vi "Main.vi"() -> ()   [LabVIEW 2014]
uses:
  Temp Sensor Folder/Global Stop TempSensor.vi
  StopForLog.vi
panel:
  out "Path":path
  out "User Name 2":string caption="שם משתמש"
  out "מספר סידורי 2":string caption="מספר סידורי"
  in  "בחירה חופשית":bool caption="Blank Button"
  in  "ממסר השהייה למפוח מפנה גזים 0410-26308":bool caption="Blank Button"
  in  "ממסר דימום מנוע 0410-26294":bool caption="Blank Button"
  in  "0410-24534 15A ממסר":bool caption="Blank Button"
  in  "0410-19646 10Ax4 ממסר":bool caption="Blank Button"
  in  "תיבת נתיכים סימן 4 0414-83040":bool caption="Blank Button"
  in  "תיבת מפעיל ריצוף 1469-98836":bool caption="Blank Button"
  in  "תיבת הזנה כיס צריח 0410-23813":bool caption="Blank Button"
  in  "Help Button":bool
  in  "Stop Button":bool
  # "צב\"ד לממסרים ונתיכים"
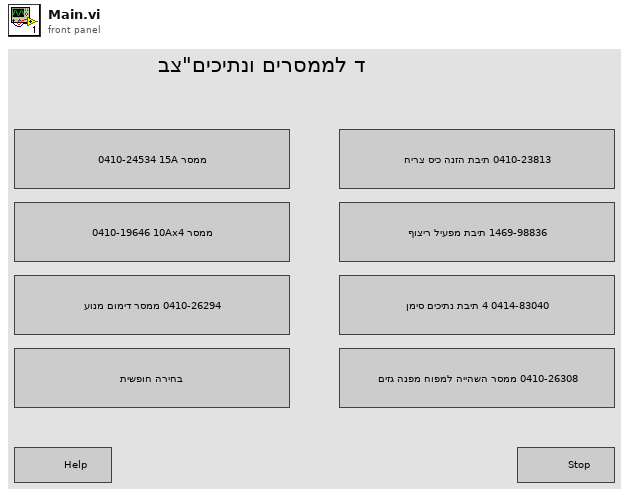
[diagram p1: front panel]
types:
  T1 = enum16{"Word Report", "User/Details", "Stop", "bhira hofshit", "ashaya mapuah mefane gazim 041026308", "dimum manoa 041026294", "memsar 4x10A 041019646", "memsar 15A 041024534", "netihim siman 4 041483040", "mafil risouf 146998836", "kis zariah 041023813", "Wait4Event", "Initialize"}
  T2 = enum16{"open", "replace", "create", "open or create", "replace or create", "replace or create with confirmation"}
  T3 = enum32{"Invalid", "Standard", "Closed", "Hidden", "Minimized", "Maximized"}
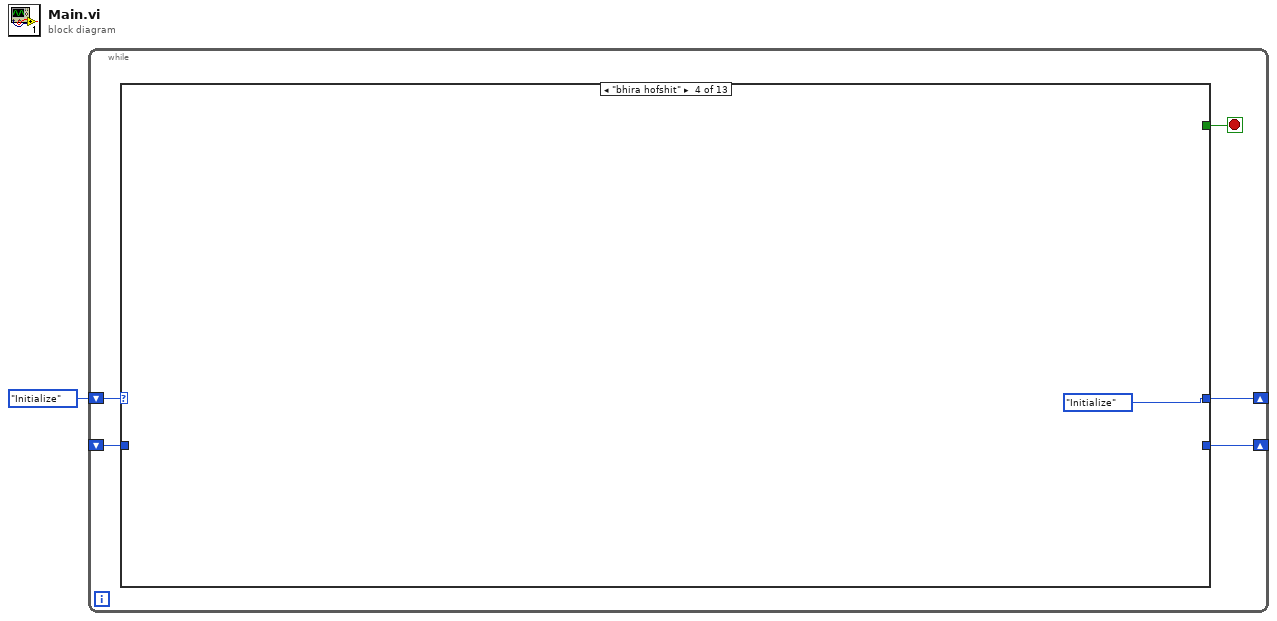
[diagram p0: block diagram]
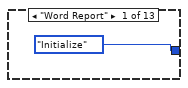
[diagram p2: hidden frame]
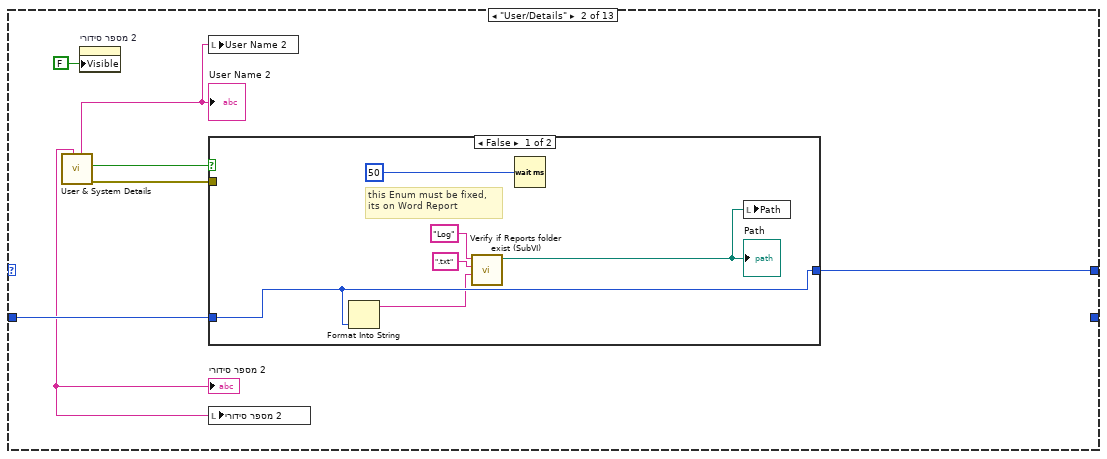
[diagram p3: hidden frame]
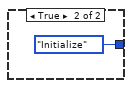
[diagram p4: hidden frame]
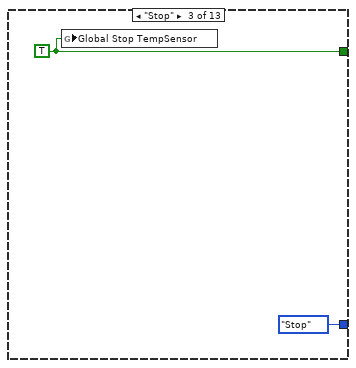
[diagram p5: hidden frame]
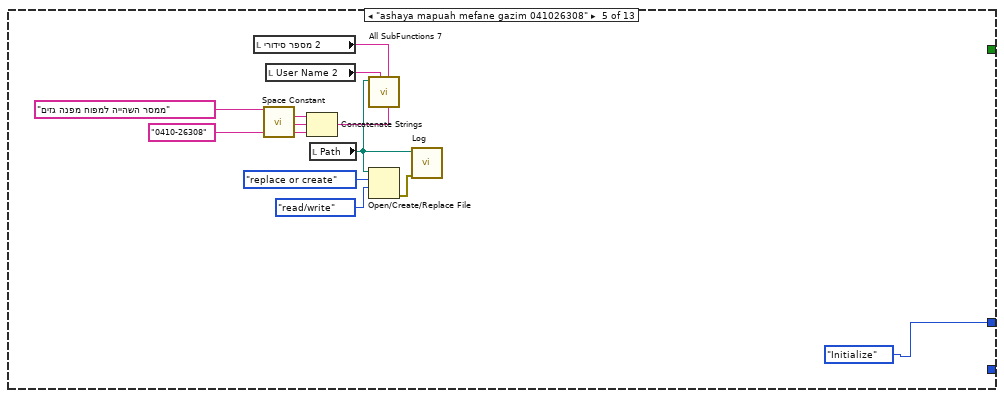
[diagram p6: hidden frame]
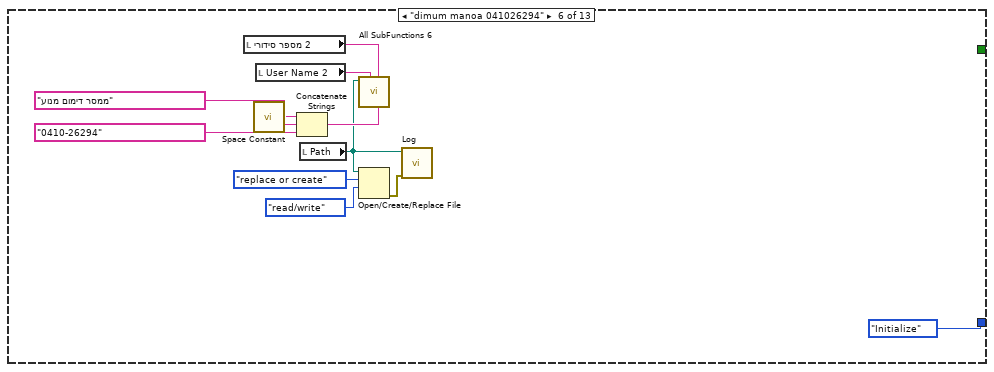
[diagram p7: hidden frame]
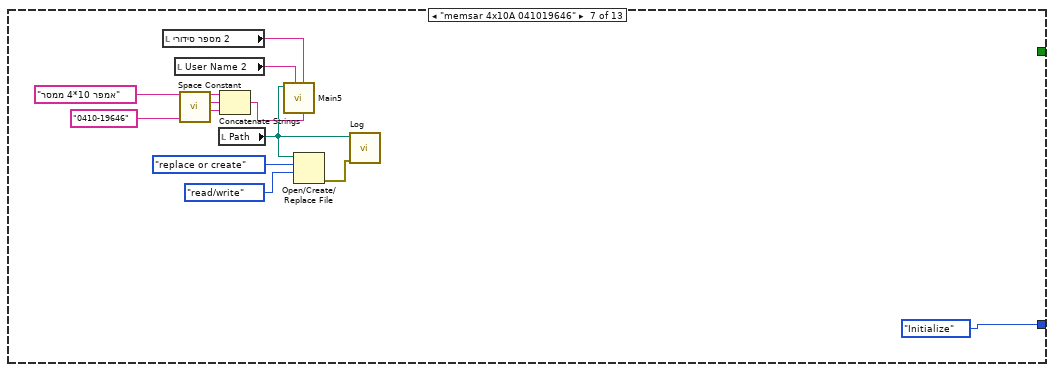
[diagram p8: hidden frame]
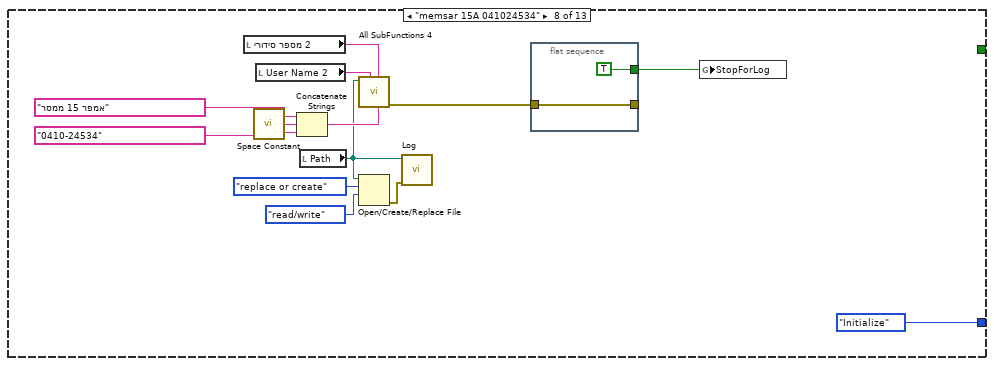
[diagram p9: hidden frame]
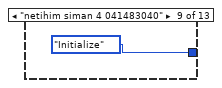
[diagram p10: hidden frame]
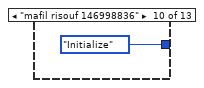
[diagram p11: hidden frame]
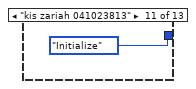
[diagram p12: hidden frame]
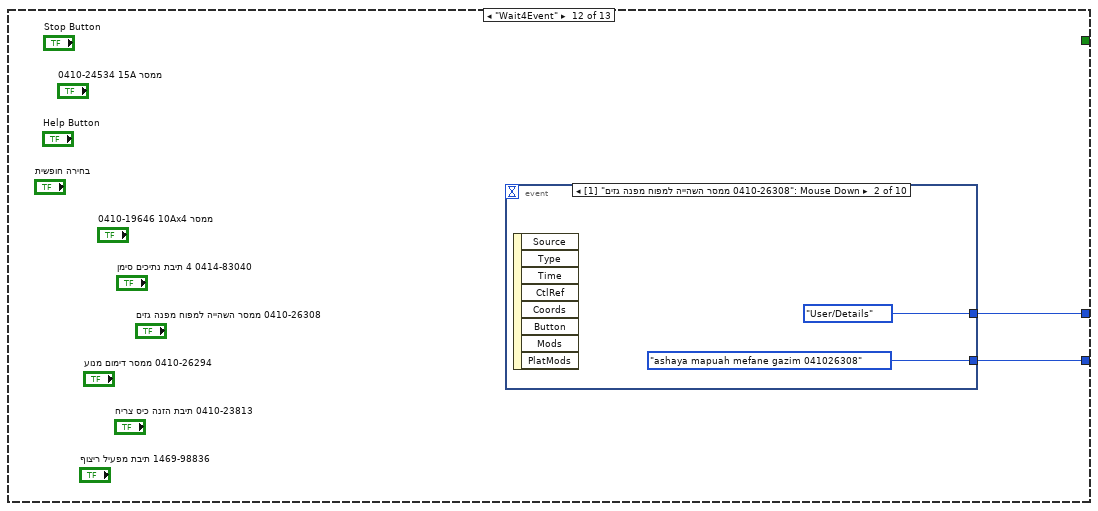
[diagram p13: hidden frame]
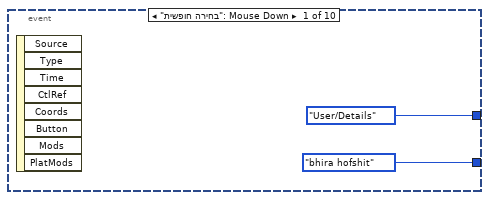
[diagram p14: hidden frame]
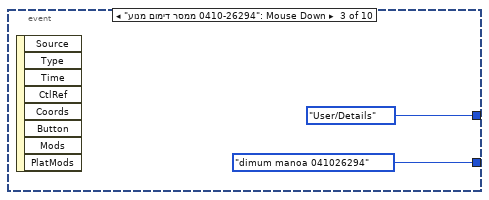
[diagram p15: hidden frame]
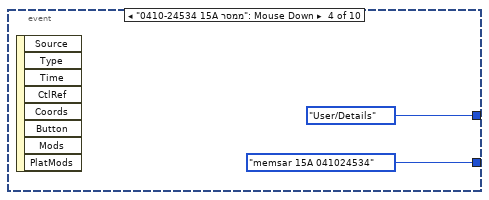
[diagram p16: hidden frame]
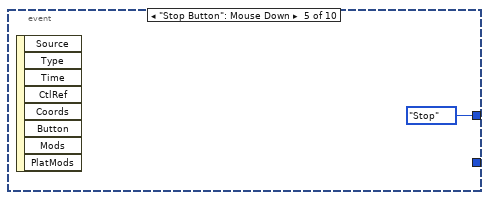
[diagram p17: hidden frame]
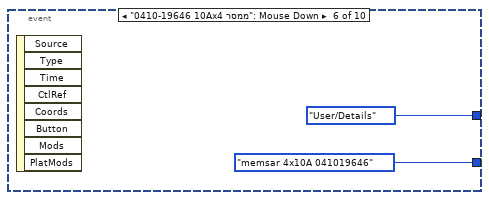
[diagram p18: hidden frame]
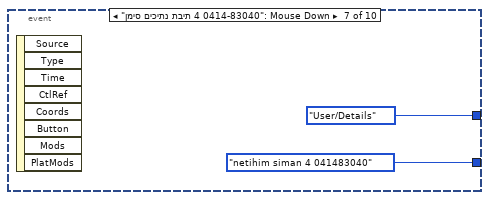
[diagram p19: hidden frame]
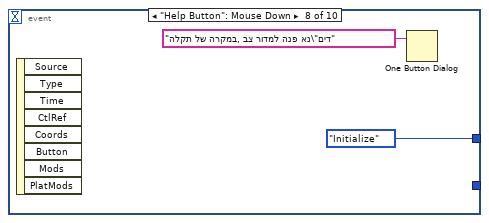
[diagram p20: hidden frame]
diagram:
  n1 = while {
    shift-right: [w5] -> _
    shift-left: T1."Initialize" -> [w6]
    shift-right: [w3] -> _
    shift-left: _ -> [w2]
    stop <- w4 stop-if-true
    n2 = case shown="\"bhira hofshit\"" w6 {
      tunnel: [T1."Initialize" w8 T1."Stop" T1."Initialize" T1."Initialize" T1."Initialize" T1."Initialize" T1."Initialize" T1."Initialize" T1."Initialize" T1."Initialize" w77 T1."Wait4Event"] -> w5
      tunnel: [_ _ w22 _ _ _ _ _ _ _ _ _ _] -> w4
      tunnel: [_ _ _ _ _ _ _ _ _ _ _ w76 _] -> w3
      tunnel: w2 -> [_ w13 _ _ _ _ _ _ _ _ _ _ _]
      frame "Word Report" {
      }
      frame "User/Details" {
        n3 = call "User & System Details.vi"() -> ("error out"=w12:errorcluster, "Boolean"=w14:bool, "User Name 2"=w9:string, "מספר סידורי 2"=w11:string)  [unwired: 8 in]
        "מספר סידורי 2" <- w11
        "User Name 2" <- w9
        n4 = property on="מספר סידורי 2" class="Str"("Visible"=FALSE) -> ()  [unwired: 2 in, 2 out]
        n5 = local write "User Name 2"(w9) -> ()
        n6 = case shown="False" w14 {
          tunnel: w13 -> [w16 _]
          tunnel: w12 -> [_ _]
          tunnel: [w16 T1."Initialize"] -> w8
          frame False {
            # "this Enum must be fixed, \nits on Word Report"
            n7 = Format Into String "Format Into String"(w16) -> (resulting string=w15:string)  [unwired: 3 in, 1 out]
            n8 = call "Verify if Reports folder exist (SubVI).vi"("שם הממסר"=w15, "File Type"=".txt", "Folder Name"="Log" ("string")) -> ("Path"=w17:path)  [unwired: 7 in, 1 out]
            "Path" <- w17
            n9 = Wait (ms)(milliseconds to wait=u32 50) -> ()  [unwired: 1 out]
            n10 = local write "Path"(w17) -> ()
          }
          frame True {
          }
        }
        n11 = local write "מספר סידורי 2"(w11) -> ()
      }
      frame "Stop" {
        w22 = TRUE
        n12 = global write "Global Stop TempSensor.vi" "Global Stop TempSensor"(w22) -> ()
      }
      frame "bhira hofshit" {
      }
      frame "ashaya mapuah mefane gazim 041026308" {
        n13 = local read "מספר סידורי 2"() -> (w31:string)
        n14 = call <vilib>:"Space Constant.vi"() -> ("String"=w34:string)
        n15 = local read "User Name 2"() -> (w32:string)
        n16 = Concatenate Strings("ממסר השהייה למפוח מפנה גזים", w34, "0410-26308") -> (w35:string)
        n17 = local read "Path"() -> (w26:path)
        n18 = call "All SubFunctions 7.vi"("מק\"ט המכלל"=w35, "מספר סידורי"=w31, "מפעיל"=w32, "Path for Log"=w26) -> ()  [unwired: 7 in, 1 out]
        n19 = Open/Create/Replace File(file path (use dialog)=w26, operation (0:open)=T2."replace or create", access (0:read/write)=enum16{"read/write", "read-only", "write-only"}."read/write") -> (error out=w27:errorcluster)  [unwired: 3 in, 2 out]
        n20 = call "Log.vi"("error in"=w27, "File Path Control"=w26) -> ()  [unwired: 8 in, 2 out]
      }
      frame "dimum manoa 041026294" {
        n21 = local read "מספר סידורי 2"() -> (w38:string)
        n22 = call <vilib>:"Space Constant.vi"() -> ("String"=w46:string)
        n23 = local read "User Name 2"() -> (w37:string)
        n24 = Concatenate Strings("ממסר דימום מנוע", w46, "0410-26294") -> (w41:string)
        n25 = local read "Path"() -> (w39:path)
        n26 = call "All SubFunctions 6.vi"("מק\"ט המכלל"=w41, "מספר סידורי"=w38, "מפעיל"=w37, "Path for Log"=w39) -> ()  [unwired: 7 in, 1 out]
        n27 = Open/Create/Replace File(file path (use dialog)=w39, operation (0:open)=T2."replace or create", access (0:read/write)=enum16{"read/write", "read-only", "write-only"}."read/write") -> (error out=w40:errorcluster)  [unwired: 3 in, 2 out]
        n28 = call "Log.vi"("error in"=w40, "File Path Control"=w39) -> ()  [unwired: 8 in, 2 out]
      }
      frame "memsar 4x10A 041019646" {
        n29 = local read "מספר סידורי 2"() -> (w48:string)
        n30 = local read "User Name 2"() -> (w49:string)
        n31 = call <vilib>:"Space Constant.vi"() -> ("String"=w55:string)
        n32 = local read "Path"() -> (w50:path)
        n33 = Concatenate Strings("ממסר 4*10 אמפר", w55, "0410-19646") -> (w52:string)
        n34 = call "Main5.vi"("מק\"ט המכלל"=w52, "מספר סידורי"=w48, "מפעיל"=w49, "Path for Log"=w50) -> ()  [unwired: 7 in, 1 out]
        n35 = Open/Create/Replace File(file path (use dialog)=w50, operation (0:open)=T2."replace or create", access (0:read/write)=enum16{"read/write", "read-only", "write-only"}."read/write") -> (error out=w51:errorcluster)  [unwired: 3 in, 2 out]
        n36 = call "Log.vi"("error in"=w51, "File Path Control"=w50) -> ()  [unwired: 8 in, 2 out]
      }
      frame "memsar 15A 041024534" {
        n37 = local read "מספר סידורי 2"() -> (w59:string)
        n38 = call <vilib>:"Space Constant.vi"() -> ("String"=w64:string)
        n39 = local read "User Name 2"() -> (w58:string)
        n40 = Concatenate Strings("ממסר 15 אמפר", w64, "0410-24534") -> (w66:string)
        n41 = local read "Path"() -> (w60:path)
        n42 = call "All SubFunctions 4.vi"("מק\"ט המכלל"=w66, "מספר סידורי"=w59, "מפעיל"=w58, "Path for Log"=w60) -> ("error IO"=w62:errorcluster)  [unwired: 7 in]
        n43 = Open/Create/Replace File(file path (use dialog)=w60, operation (0:open)=T2."replace or create", access (0:read/write)=enum16{"read/write", "read-only", "write-only"}."read/write") -> (error out=w63:errorcluster)  [unwired: 3 in, 2 out]
        n44 = call "Log.vi"("error in"=w63, "File Path Control"=w60) -> ()  [unwired: 8 in, 2 out]
        n45 = flat-sequence {
          tunnel: w62 -> [w71]
          tunnel: [TRUE] -> w61
          tunnel: [w71] -> _
          frame #0 {
          }
        }
        n46 = global write "StopForLog.vi" "StopForLog"(w61) -> ()
      }
      frame "netihim siman 4 041483040" {
      }
      frame "mafil risouf 146998836" {
      }
      frame "kis zariah 041023813" {
      }
      frame "Wait4Event" {
        n47 = event shown="[1] \"ממסר השהייה למפוח מפנה גזים 0410-26308\": Mouse Down" {
          selector: _ -> [_ _ _ _ _ _ _ _ _ _]
          dyn-events: _ -> [_ _ _ _ _ _ _ _ _ _]
          timeout: _ -> [_ _ _ _ _ _ _ _ _ _]
          tunnel: [T1."User/Details" T1."User/Details" T1."User/Details" T1."User/Details" T1."Stop" T1."User/Details" T1."User/Details" T1."Initialize" T1."User/Details" T1."User/Details"] -> w77
          tunnel: [T1."bhira hofshit" T1."ashaya mapuah mefane gazim 041026308" T1."dimum manoa 041026294" T1."memsar 15A 041024534" _ T1."memsar 4x10A 041019646" T1."netihim siman 4 041483040" _ T1."mafil risouf 146998836" T1."kis zariah 041023813"] -> w76
          event "בחירה חופשית": Mouse Down {
            n48 = event-data() -> ()  [unwired: 1 in, 8 out]
          }
          event "ממסר השהייה למפוח מפנה גזים 0410-26308": Mouse Down {
            n49 = event-data() -> ()  [unwired: 1 in, 8 out]
          }
          event "ממסר דימום מנוע 0410-26294": Mouse Down {
            n50 = event-data() -> ()  [unwired: 1 in, 8 out]
          }
          event "0410-24534 15A ממסר": Mouse Down {
            n51 = event-data() -> ()  [unwired: 1 in, 8 out]
          }
          event "Stop Button": Mouse Down {
            n52 = event-data() -> ()  [unwired: 1 in, 8 out]
          }
          event "0410-19646 10Ax4 ממסר": Mouse Down {
            n53 = event-data() -> ()  [unwired: 1 in, 8 out]
          }
          event "תיבת נתיכים סימן 4 0414-83040": Mouse Down {
            n54 = event-data() -> ()  [unwired: 1 in, 8 out]
          }
          event "Help Button": Mouse Down {
            n55 = event-data() -> ()  [unwired: 1 in, 8 out]
            n56 = One Button Dialog(message="במקרה של תקלה, נא פנה למדור צב\"דים") -> ()  [unwired: 1 in, 1 out]
          }
          event "תיבת מפעיל ריצוף 1469-98836": Mouse Down {
            n57 = event-data() -> ()  [unwired: 1 in, 8 out]
          }
          event "תיבת הזנה כיס צריח 0410-23813": Mouse Down {
            n58 = event-data() -> ()  [unwired: 1 in, 8 out]
          }
        }
      }
      frame "Initialize", Default {
        n59 = vi-ref "Main.vi"() -> (w99:refnum<vi>)
        n60 = global write "Global Stop TempSensor.vi" "Global Stop TempSensor"(FALSE ("Global Stop TempSensor")) -> ()
        n61 = property class="VI"(reference=w99) -> (reference out=w98:refnum<vi>, "FP.State"=w97:T3)  [unwired: 1 in, 1 out]
        n62 = case shown="\"Closed\"" w97 {
          tunnel: w98 -> [w111 w113 w117 w119 w123 w125]
          frame "Invalid", Default {
            n63 = invoke class="VI" method="FP.Open"(reference=w111, "Activate"=FALSE ("Wait Until Done"), "State"=T3."Standard") -> ()  [unwired: 2 in, 5 out]
          }
          frame "Standard" {
            n64 = invoke class="VI" method="FP.Open"(reference=w113, "Activate"=FALSE ("Wait Until Done"), "State"=T3."Standard") -> ()  [unwired: 2 in, 5 out]
          }
          frame "Closed" {
            n65 = invoke class="VI" method="FP.Open"(reference=w117, "Activate"=FALSE ("Wait Until Done"), "State"=T3."Standard") -> ()  [unwired: 2 in, 5 out]
          }
          frame "Hidden" {
            n66 = invoke class="VI" method="FP.Open"(reference=w119, "Activate"=FALSE ("Wait Until Done"), "State"=T3."Standard") -> ()  [unwired: 2 in, 5 out]
          }
          frame "Minimized" {
            n67 = invoke class="VI" method="FP.Open"(reference=w123, "Activate"=FALSE ("Wait Until Done"), "State"=T3."Standard") -> ()  [unwired: 2 in, 5 out]
          }
          frame "Maximized" {
            n68 = invoke class="VI" method="FP.Open"(reference=w125, "Activate"=FALSE ("Wait Until Done"), "State"=T3."Standard") -> ()  [unwired: 2 in, 5 out]
          }
        }
        n69 = call <vilib>:"Application Directory.vi"() -> ("Application Directory"=w108:path)
        n70 = Build Path(base path=w108, name or relative path="Temp Sensor Folder\\Temp Sensor.vi") -> (appended path=w106:path)
        n71 = Open VI Reference(vi path=w106) -> (vi reference=w105:refnum<vi>, error out=w104:errorcluster)  [unwired: 5 in]
        n72 = property class="VI"(reference=w105, error in=w104) -> (reference out=w101:refnum<vi>, error out=w102:errorcluster, "FP.State"=w103:T3)
        n73 = case shown="\"Invalid\", Default" w103 {
          tunnel: w102 -> [w129 w136 w142 _ _ _]
          tunnel: w101 -> [w128 w135 w143 _ _ _]
          frame "Invalid", Default {
            w134 = FALSE ("Wait Until Done")
            n74 = invoke class="VI" method="FP.Open"(reference=w128, error in=w129, "Activate"=w134, "State"=T3."Minimized") -> (reference out=w131:refnum<vi>, error out=w132:errorcluster)  [unwired: 1 in, 3 out]
            n75 = invoke class="VI" method="Run VI"(reference=w131, error in=w132, "Wait until done"=w134, "Auto Dispose Ref"=FALSE ("Auto Dispose Reference")) -> ()  [unwired: 1 in, 5 out]
          }
          frame "Standard" {
            w141 = FALSE ("Wait Until Done")
            n76 = invoke class="VI" method="FP.Open"(reference=w135, error in=w136, "Activate"=w141, "State"=T3."Minimized") -> (reference out=w138:refnum<vi>, error out=w139:errorcluster)  [unwired: 1 in, 3 out]
            n77 = invoke class="VI" method="Run VI"(reference=w138, error in=w139, "Wait until done"=w141, "Auto Dispose Ref"=FALSE ("Auto Dispose Reference")) -> ()  [unwired: 1 in, 5 out]
          }
          frame "Closed" {
            w148 = FALSE ("Wait Until Done")
            n78 = invoke class="VI" method="FP.Open"(reference=w143, error in=w142, "Activate"=w148, "State"=T3."Minimized") -> (reference out=w145:refnum<vi>, error out=w146:errorcluster)  [unwired: 1 in, 3 out]
            n79 = invoke class="VI" method="Run VI"(reference=w145, error in=w146, "Wait until done"=w148, "Auto Dispose Ref"=FALSE ("Auto Dispose Reference")) -> ()  [unwired: 1 in, 5 out]
          }
          frame "Hidden" {
          }
          frame "Minimized" {
          }
          frame "Maximized" {
          }
        }
      }
    }
  }
